vi "Licor-Commands (source).vi"(0 "type":string, 2 "response?":bool, 7 "value":string) -> (8 "out":string)   [LabVIEW 2010]
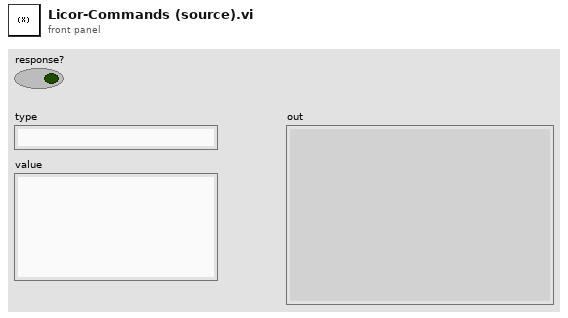
[diagram p1: front panel]
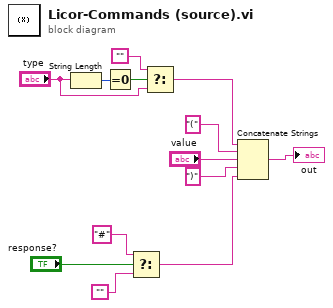
[diagram p0: block diagram]
diagram:
  n1 = String Length(string="type") -> (length=w9:i32)
  n2 = Equal To 0?(x=w9) -> (x = 0?=w8:bool)
  n3 = Select(t="#", s="response?", f="") -> (s? t:f=w1:string)
  n4 = Select(t="", s=w8, f="type") -> (s? t:f=w5:string)
  n5 = Concatenate Strings(w5, "(", "value", ")", w1) -> (→"out":string)
